vi "labscope.vi"() -> ()   [LabVIEW 2016]
uses:
  <vilib>/Utility/error.llb/DialogType.ctl
  <vilib>/express/express analysis/Spectral/Block/exnSpectralBlock spectral measurements RMS poly.vi
  <vilib>/express/express analysis/Spectral/Block/exnSpectralBlock spectral measurements RMS WFM.vi
  <vilib>/express/express analysis/Spectral/XNode/ExpressSpectralMeasurementsBlockNode.xnode
panel:
  out "Spectrum":cluster{"f0":dbl, "df":dbl, "magnitude":dbl[]}(graph)
  in  "Session Name":string="pe510k1"
  in  "stop":bool
  out "Waveform":dbl[](graph)
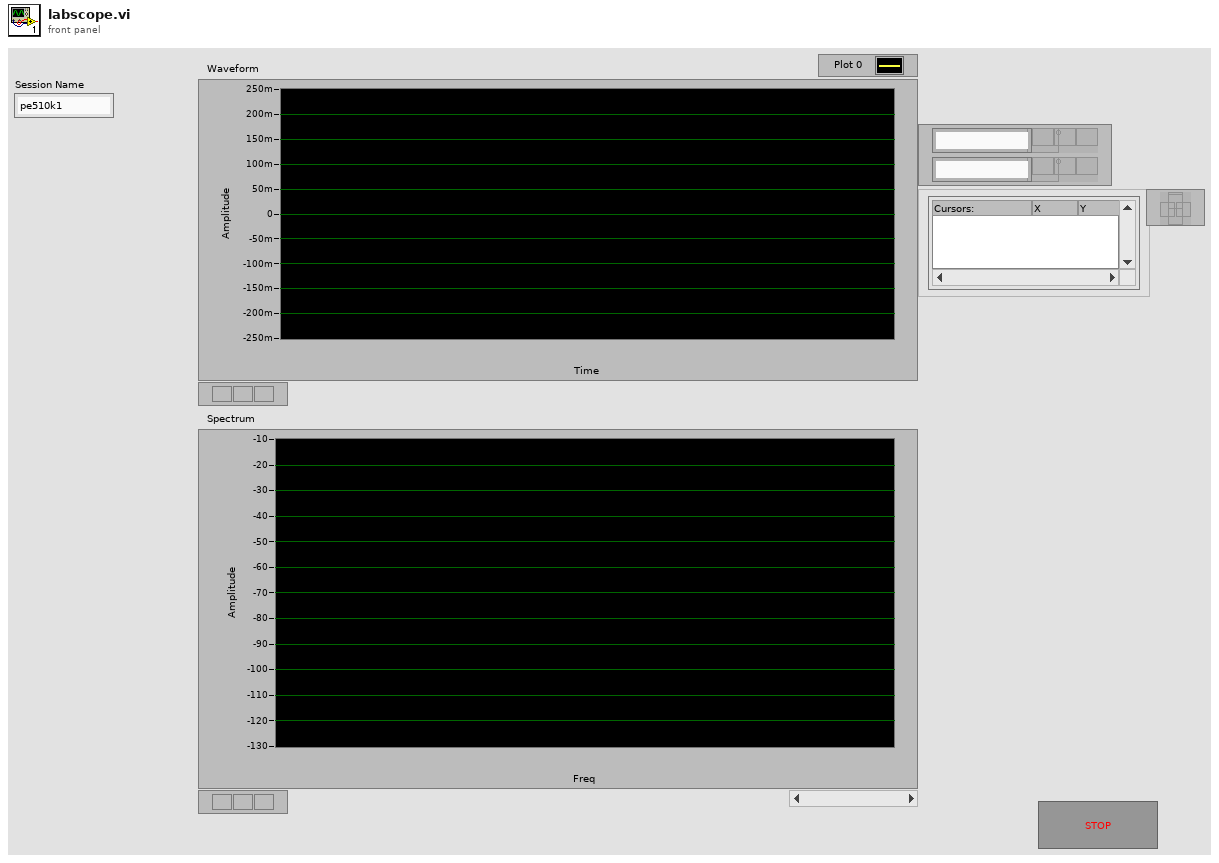
[diagram p1: front panel]
types:
  T1 = typedef "DialogType.ctl" = u16
  T2 = cluster{"averaging mode":u16, "weighting mode":u16, "number of averages":u32}
  T3 = cluster{"dB On (F)":bool, "unwrap phase (F)":bool, "convert to degree (F)":bool}
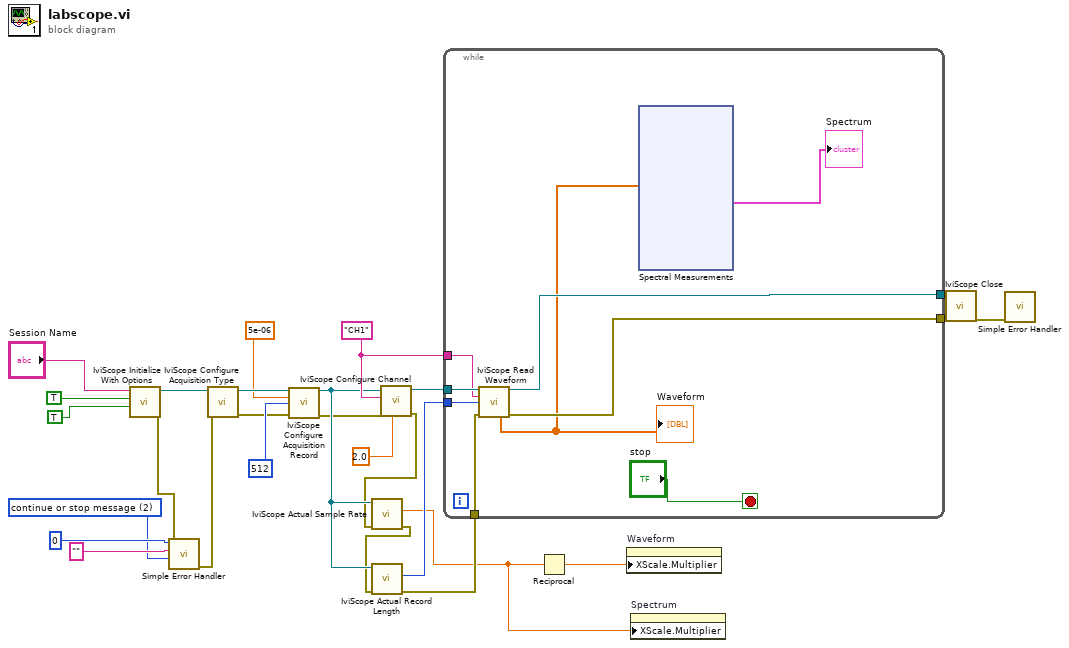
[diagram p0: block diagram]
diagram:
  w3 = T1 2 items=["no dialog", "OK message", "continue or stop message", "OK message + warnings", "continue/stop + warnings"] ("type of dialog (OK msg:1)")
  w20 = "CH1"
  n1 = call <vilib>:"IviScope Initialize With Options.vi"("reset device (True)"=TRUE, "id query (True)"=TRUE, "logical name (\"SampleScope\")"="Session Name") -> ("error out"=w7:errorcluster, "instrument handle out"=w25:refnum<k15>)  [unwired: 7 in]
  n2 = call <vilib>:"Simple Error Handler.vi"("error code (no error:0)"=0, "error source (\" \")"="" ("error source (\" \")"), "type of dialog (OK msg:1)"=w3, "error in (no error)"=w7) -> ("error out"=w6:errorcluster)  [unwired: 1 in, 4 out]
  n3 = call <vilib>:"IviScope Configure Acquisition Type.vi"("error in (no error)"=w6, "instrument handle"=w25) -> ("error out"=w13:errorcluster, "instrument handle out"=w24:refnum<k15>)  [unwired: 8 in]
  n4 = call <vilib>:"IviScope Configure Acquisition Record.vi"("instrument handle"=w24, "time per record (1.0E-3 s)"=5e-06, "min record length (100 samples)"=512, "error in (no error)"=w13) -> ("instrument handle out"=w17:refnum<k15>, "error out"=w12:errorcluster)  [unwired: 10 in]
  n5 = call <vilib>:"IviScope Configure Channel.vi"("vertical range (10.0 V)"=2.0, "error in (no error)"=w12, "channel name (\"CHANNEL1\")"=w20, "instrument handle"=w17) -> ("error out"=w11:errorcluster, "instrument handle out"=w18:refnum<k15>)  [unwired: 6 in]
  n6 = call <vilib>:"IviScope Actual Sample Rate.vi"("error in (no error)"=w11, "instrument handle"=w17) -> ("error out"=w10:errorcluster, "sample rate"=w1:dbl)  [unwired: 7 in, 1 out]
  n7 = call <vilib>:"IviScope Actual Record Length.vi"("error in (no error)"=w10, "instrument handle"=w17) -> ("error out"=w9:errorcluster, "actual record length"=w16:i32)  [unwired: 7 in, 1 out]
  n8 = while {
    tunnel: w18 -> [w36]
    tunnel: w20 -> [w35]
    tunnel: [w33] -> w19
    tunnel: w16 -> [w32]
    tunnel: w9 -> [w31]
    tunnel: [w30] -> w2
    stop <- "stop" stop-if-true
    n9 = call <vilib>:"IviScope Read Waveform.vi"("instrument handle"=w36, "channel name (\"CHANNEL1\")"=w35, "waveform size (0)"=w32, "error in (no error)"=w31) -> ("instrument handle out"=w33:refnum<k15>, "waveform array"=w29:dbl[], "error out"=w30:errorcluster)  [unwired: 6 in, 3 out]
    "Waveform" <- w29
    n10 = xnode "Spectral Measurements"("Signals"=w29) -> ("FFT - (RMS)"=→"Spectrum":cluster{"f0":dbl, "df":dbl, "magnitude":dbl[]})  [unwired: 1 in, 2 out]
  }
  n11 = Reciprocal(x=w1) -> (1/x=w15:dbl)
  n12 = property on="Waveform" class="WFGraph (strict)"("XScale.Multiplier"=w15) -> ()  [unwired: 2 in, 2 out]
  n13 = property on="Spectrum" class="WFGraph (strict)"("XScale.Multiplier"=w1) -> ()  [unwired: 2 in, 2 out]
  n14 = call <vilib>:"IviScope Close.vi"("error in (no error)"=w2, "instrument handle"=w19) -> ("error out"=w8:errorcluster)  [unwired: 9 in]
  n15 = call <vilib>:"Simple Error Handler.vi"("error in (no error)"=w8) -> ()  [unwired: 4 in, 5 out]
